vi "plus and minus (dbl).vi"(9 "b":dbl, 10 "a":dbl) -> (1 "a-b":dbl, 2 "a+b":dbl)   [LabVIEW 2013]
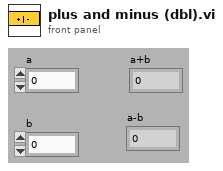
[diagram p1: front panel]
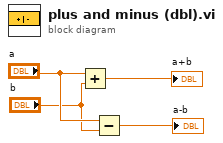
[diagram p0: block diagram]
diagram:
  n1 = Add(x="a", y="b") -> (x+y=→"a+b":dbl)
  n2 = Subtract(x="a", y="b") -> (x-y=→"a-b":dbl)
